vi "AC_Source_IDRC.vi"(8 "error_in":errorcluster, 9 "Parameter":T1, 10 "Mode":T2(ring)=enum."TurnOn", 11 "GPIB Address":string) -> (0 "error_out":errorcluster, 3 "Response":string)   [LabVIEW 2019]
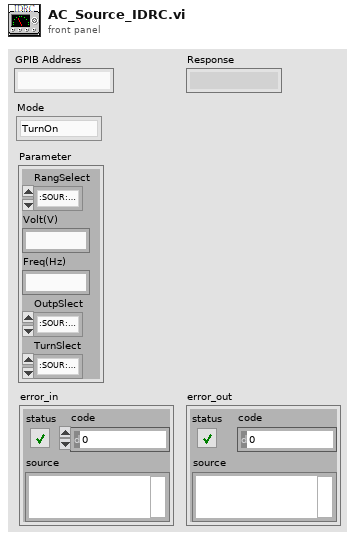
[diagram p1: front panel]
types:
  T1 = cluster{"RangSelect":enum16{":SOUR:RANG LOW;", ":SOUR:RANG HIGH;", ":SOUR:RANG AUTO;"}, "Volt(V)":string, "Freq(Hz)":string, "OutpSlect":enum16{":SOUR:TURN OFF;", ":SOUR:TURN ON;"}, "TurnSlect":enum16{":SOUR:TURN OFF;", ":SOUR:TURN ON;"}}
  T2 = enum16{"SetRange", "SetVoltage", "SetFreq", "OUTP", "TurnOn"}
  T3 = enum16{":SOUR:RANG LOW;", ":SOUR:RANG HIGH;", ":SOUR:RANG AUTO;"}
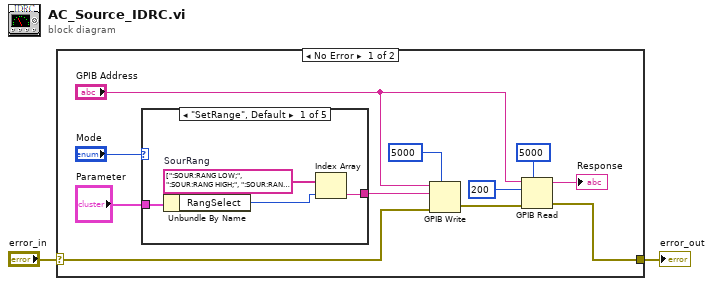
[diagram p0: block diagram]
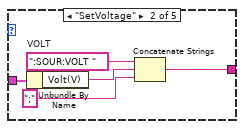
[diagram p2: hidden frame]
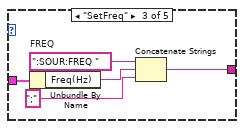
[diagram p3: hidden frame]
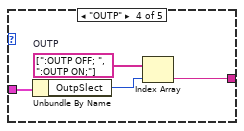
[diagram p4: hidden frame]
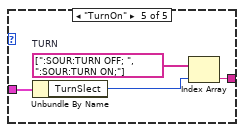
[diagram p5: hidden frame]
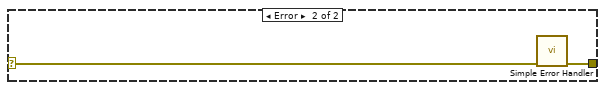
[diagram p6: hidden frame]
diagram:
  n1 = case shown="No Error" "error_in" {
    selector: "error_in" -> [w4 w37]
    tunnel: [w3 w36] -> w1
    frame No Error {
      n2 = case shown="\"SetRange\", Default" "Mode" {
        tunnel: "Parameter" -> [w16 w20 w25 w30 w34]
        tunnel: [w14 w18 w23 w29 w32] -> w5
        frame "SetRange", Default {
          w17 = string[] [":SOUR:RANG LOW;", ":SOUR:RANG HIGH;", ":SOUR:RANG AUTO;"]  # SourRang
          n3 = Unbundle By Name(w16) -> ("RangSelect"=w15:T3)
          n4 = Index Array(array=w17, index=w15) -> (element=w14:string)
        }
        frame "SetVoltage" {
          w22 = ":SOUR:VOLT "  # VOLT
          n5 = Unbundle By Name(w20) -> ("Volt(V)"=w19:string)
          n6 = Concatenate Strings(w22, w19, ";" ("string")) -> (w18:string)
        }
        frame "SetFreq" {
          w27 = ":SOUR:FREQ "  # FREQ
          n7 = Unbundle By Name(w25) -> ("Freq(Hz)"=w24:string)
          n8 = Concatenate Strings(w27, w24, ";" ("string")) -> (w23:string)
        }
        frame "OUTP" {
          w31 = string[] [":OUTP OFF; ", ":OUTP ON;"]  # OUTP
          n9 = Unbundle By Name(w30) -> ("OutpSlect"=w28:enum16{":SOUR:TURN OFF;", ":SOUR:TURN ON;"})
          n10 = Index Array(array=w31, index=w28) -> (element=w29:string)
        }
        frame "TurnOn" {
          w35 = string[] [":SOUR:TURN OFF; ", ":SOUR:TURN ON;"]  # TURN
          n11 = Unbundle By Name(w34) -> ("TurnSlect"=w33:enum16{":SOUR:TURN OFF;", ":SOUR:TURN ON;"})
          n12 = Index Array(array=w35, index=w33) -> (element=w32:string)
        }
      }
      n13 = GPIB Write(0:"GPIB Address", 1:w5, 3:w4, 4:5000 ("timeout (ms)")) -> (6:w12:errorcluster)  [unwired: 1 in, 1 out]
      n14 = GPIB Read(0:"GPIB Address", 1:200 ("byte count"), 3:w12, 4:5000 ("timeout (ms)")) -> (5:→"Response":string, 7:w3:errorcluster)  [unwired: 1 in, 1 out]
    }
    frame Error {
      n15 = call <vilib>:"Simple Error Handler.vi"("error in (no error)"=w37) -> ("error out"=w36:errorcluster)  [unwired: 4 in, 4 out]
    }
  }
  "error_out" <- w1
